vi "CH_LM DFM Delete File.vi"(0 "Meter Index":i32, 1 "Type":bool, 2 "Directory or File Name (\"\")":string, 5 "error in (no error)":errorcluster, 7 "Timeout / ms (3000)":i32=3000, 9 "Lock Timeout / ms (1000)":i32=1000) -> (11 "Lock timed out":bool, 14 "Meter Index":i32, 19 "error out":errorcluster)   [LabVIEW 2012, in "CH_LM.lvlib"]
doc: "This command will delete a file or remove a directory.\n\n<B>Attention:</B> An attempt to delete a non-existent file will raise error 201. An attempt to delete a file being populated by the currently active trend cycle will raise error 101. An attempt to delete a file open for file transfer will raise error 101. An attempt to remove a directory that does not exist will raise error 200. An attempt to remove a directory that contains files or subdirectories will raise error 204."
uses:
  CH_LM.lvlib
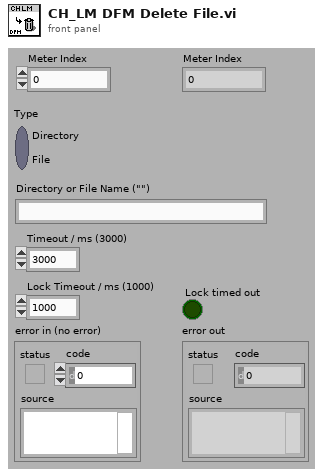
[diagram p1: front panel]
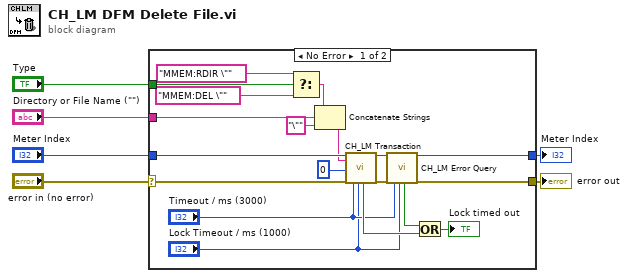
[diagram p0: block diagram]
diagram:
  n1 = case shown="No Error" "error in (no error)" {
    selector: "error in (no error)" -> [w25 w27]
    tunnel: [w22 w27] -> w6
    tunnel: "Meter Index" -> [w24 w26]
    tunnel: [w23 w26] -> w3
    tunnel: "Directory or File Name (\"\")" -> [w21 _]
    tunnel: "Type" -> [w7 _]
    frame No Error {
      n2 = Select(t="MMEM:RDIR \"" ("Command String"), s=w7, f="MMEM:DEL \"" ("Command String")) -> (s? t:f=w8:string)
      n3 = Concatenate Strings(w8, w21, "\"" ("string")) -> (w12:string)
      n4 = call "CH_LM Transaction.vi"("Meter Index"=w24, "Command String"=w12, "NofStrings (-1:all)"=0 ("t"), "error in (no error)"=w25, "Timeout / ms (3000)"="Timeout / ms (3000)", "Lock Timeout / ms (1000)"="Lock Timeout / ms (1000)") -> ("Lock timed out"=w16:bool, "Meter Index"=w19:i32, "error out"=w18:errorcluster)  [unwired: 11 out]
      n5 = call "CH_LM Error Query.vi"("Meter Index"=w19, "error in (no error)"=w18, "Timeout / ms (3000)"="Timeout / ms (3000)", "Lock Timeout / ms (1000)"="Lock Timeout / ms (1000)") -> ("Lock timed out"=w17:bool, "Meter Index"=w23:i32, "error out"=w22:errorcluster)  [unwired: 13 out]
      n6 = Or(x=w17, y=w16) -> (x .or. y?=→"Lock timed out":bool)
    }
    frame Error {
    }
  }
  "error out" <- w6
  "Meter Index" <- w3
